vi "lsl pull sample buf.vi"(0 "in":cluster{}, 1 "timeout":dbl, 5 "buffer":string, 7 "buffer_lengths":u32, 9 "buffer_elements":i32, 11 "error in (no error)":errorcluster, 12 "ec":i32) -> (4 "in out":cluster{}, 6 "buffer out":string, 8 "buffer_lengths out":u32, 10 "function return":dbl, 14 "ec out":i32, 15 "error out":errorcluster)   [LabVIEW 2018, in "liblsl-LabVIEW.lvlib"]
doc: "extern LIBLSL_C_API double lsl_pull_sample_buf(lsl_inlet in, char **buffer, uint32_t *buffer_lengths, int32_t buffer_elements, double timeout, int32_t *ec);"
uses:
  <userlib>/liblsl-LabVIEW/liblsl-LabVIEW.lvlib
  <userlib>/liblsl-LabVIEW/liblsl64.dll
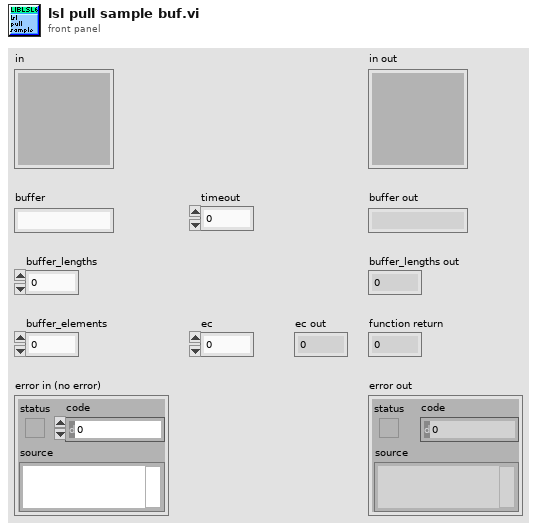
[diagram p1: front panel]
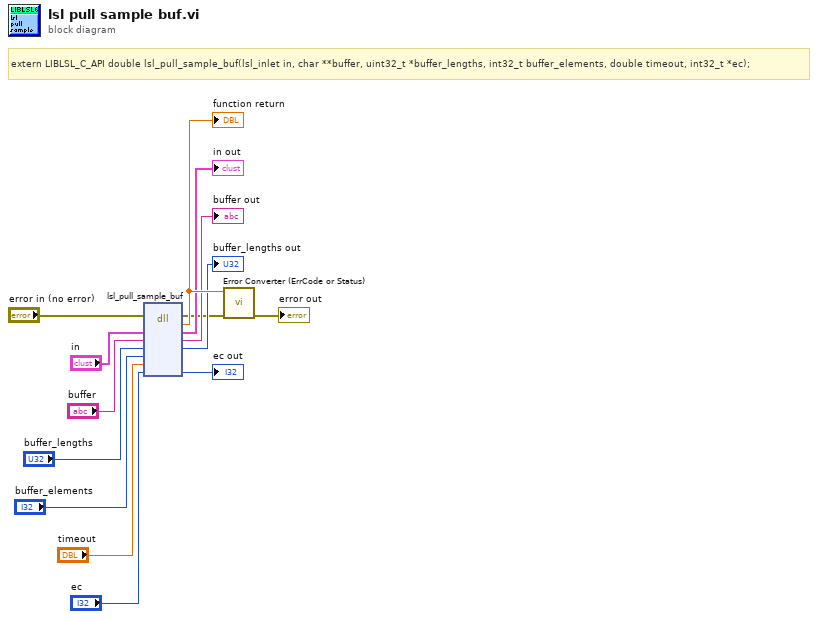
[diagram p0: block diagram]
diagram:
  # "extern LIBLSL_C_API double lsl_pull_sample_buf(lsl_inlet in, char **buffer, uint32_t *buffer_lengths, int32_t buffer_elements, double timeout, int32_t *ec);"
  n1 = dll-call lib="C:/Program Files/National Instruments/LabVIEW 2018/user.lib/liblsl-LabVIEW/liblsl64.*" fn="lsl_pull_sample_buf"(error in="error in (no error)", "in"="in", "buffer"="buffer", "buffer_lengths"="buffer_lengths", "buffer_elements"="buffer_elements", "timeout"="timeout", "ec"="ec") -> (error out=w2:errorcluster, w14:dbl, "in"=→"in out":cluster{}, "buffer"=→"buffer out":string, "buffer_lengths"=→"buffer_lengths out":u32, "ec"=→"ec out":i32)  [unwired: 4 in, 1 out]
  "function return" <- w14
  n2 = call <userlib>:"Error Converter (ErrCode or Status).vi"("error in (no error)"=w2, "error code"=w14) -> ("error out"=→"error out":errorcluster)  [unwired: 9 in]
